vi "ResMgr-BackgroundThread.vi"(7 "Name (Unnamed)":string) -> ()   [LabVIEW 2017, in "Communicable State Machine.lvlib"]
uses:
  Communicable State Machine.lvlib
  Typedef/_CSM_GlobalLog_MSG.ctl
  Typedef/_CSM_Response Source Message.ctl
  Typedef/_CSM_GlobalLog_MSG_TYPE.ctl
  CSMQ/_CSMObj-ModeData.ctl
  CSMQ/_CSMObj-Data.ctl
  Typedef/_CSM_MSG_TYPE.ctl
  Priority Queue/Priority Queue.ctl
  Typedef/_Cross CSM State Data.ctl
  Typedef/_Cross CSM State Response.ctl
  Priority Queue/def-Data(LowPRI-Q).ctl
  Typedef/_CSM Status Change Event Data.ctl
panel:
  out "Array":string[](array[string])
  out "size(s)":i32
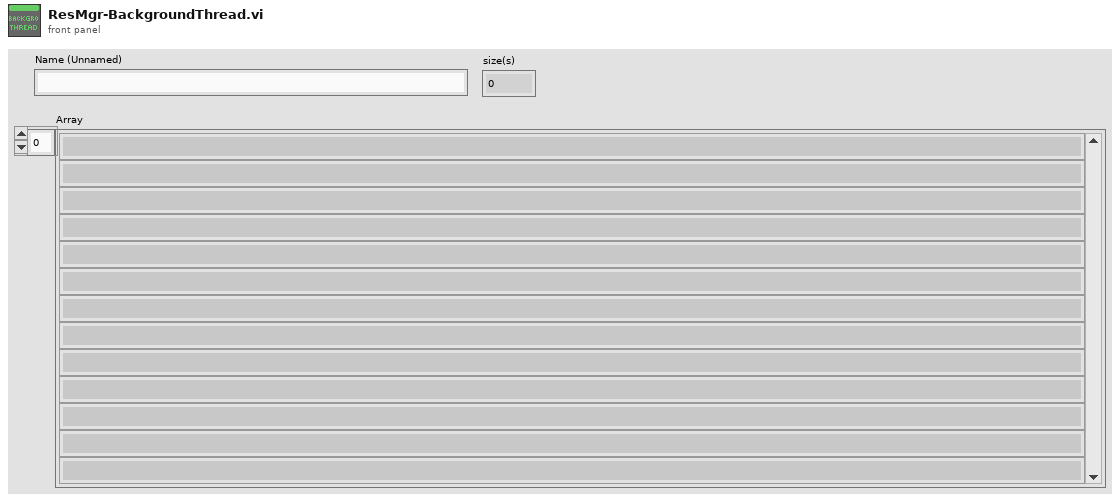
[diagram p1: front panel]
types:
  T1 = typedef "Communicable State Machine.lvlib/_CSM_GlobalLog_MSG.ctl" = cluster{"Name (\"\" to Use UUID)":string, "Current State":string, "Arguments":string, "Source Message":T2, "Source Module":string, "Complete(T)/Start(F)":bool, "LogType":T3, "Time Stamp":timestamp}
  T2 = typedef "Communicable State Machine.lvlib/_CSM_Response Source Message.ctl" = cluster{"‘State":string, "’Arguments":string, "’Error":errorcluster}
  T3 = typedef "Communicable State Machine.lvlib/_CSM_GlobalLog_MSG_TYPE.ctl" = enum16{"User Log", "State Change", "Status", "Interrupt", "Register", "Unregister", "Error Log", "Module Created", "Module Destroyed", "Async Message", "No-Rep Async Message", "Sync Message"}
  T4 = typedef "Communicable State Machine.lvlib/_CSMObj-ModeData.ctl" = cluster{"CSMDataDVR":refnum<data-value>[], "PriorityQueues":T5[], "Messages of Chain Nodes":cluster{"Module Name":string, "Allowed Messages":string[]}[], "Chain Message Mapping Map":variant, "SharedRegistryRules":string[]}
  T5 = typedef "Communicable State Machine.lvlib/Priority Queue.ctl" = cluster{"HPriorityQ":refnum<queue>, "LowPriorityQ":refnum<queue>}
  T6 = typedef "Communicable State Machine.lvlib/_CSM Status Change Event Data.ctl" = cluster{"ModuleName":string, "Status":string, "Arguments":string}
  T7 = cluster{"ResType":string, "RespQ":refnum<queue>, "Parameter":string, "WatchDogQ":refnum<queue>}
  T8 = cluster{"Major":u16, "Minor":u16, "Fix":u16, "Build":u16}
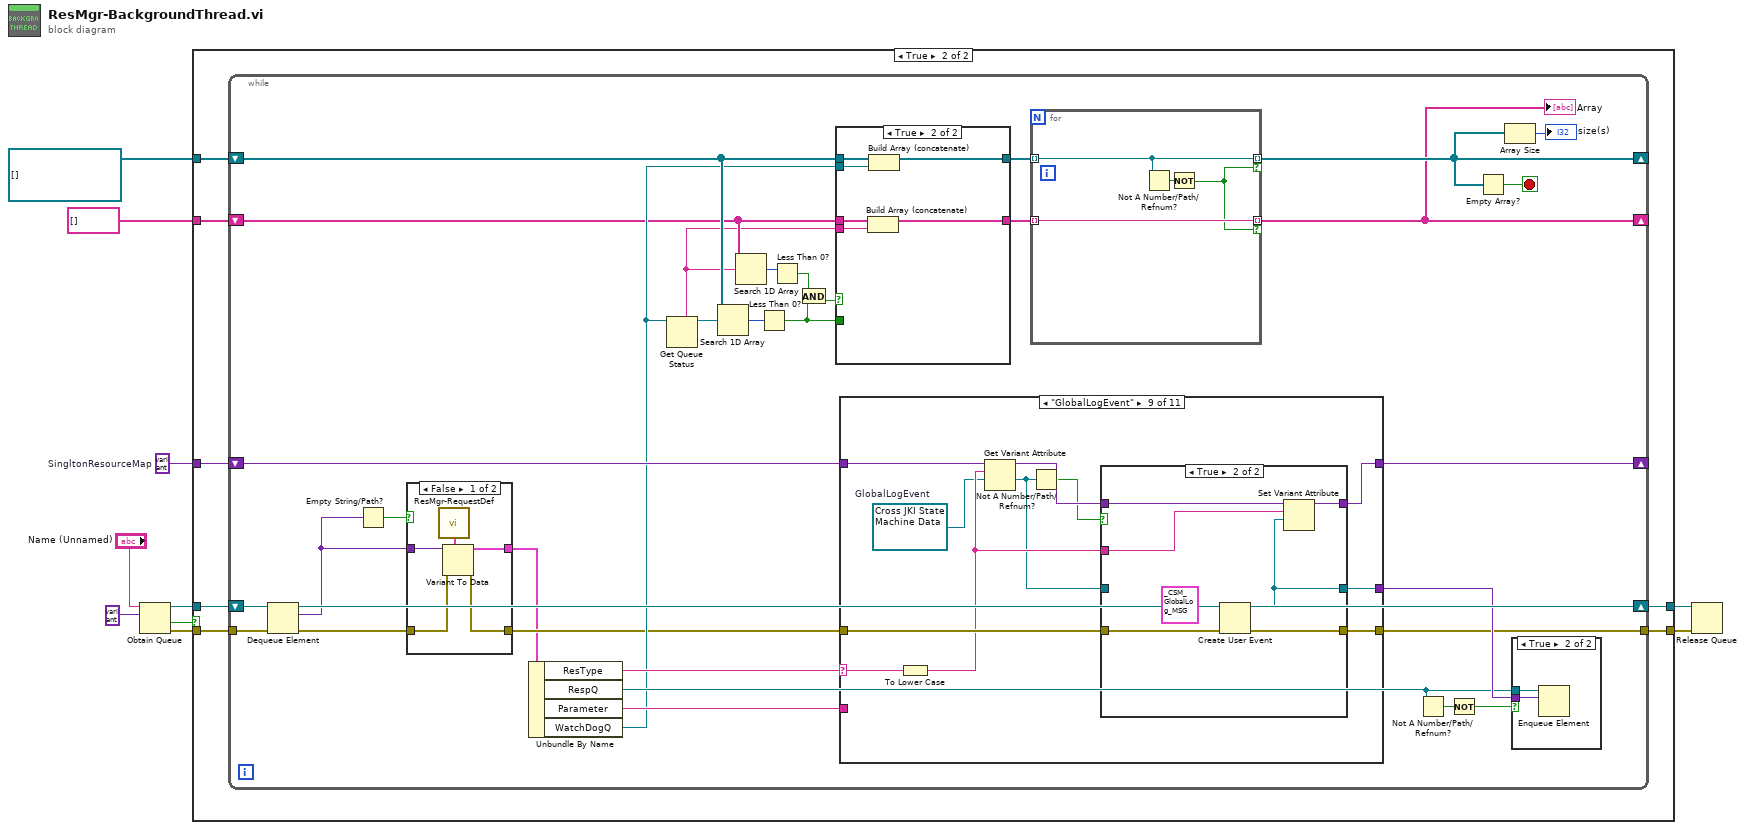
[diagram p0: block diagram]
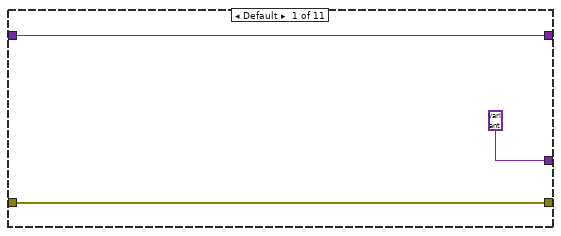
[diagram p6: hidden frame]
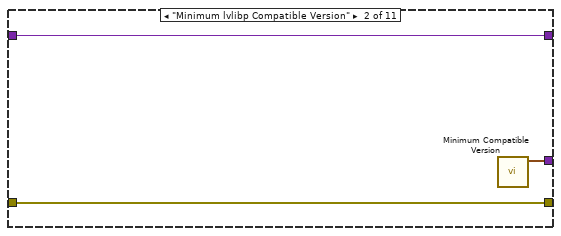
[diagram p7: hidden frame]
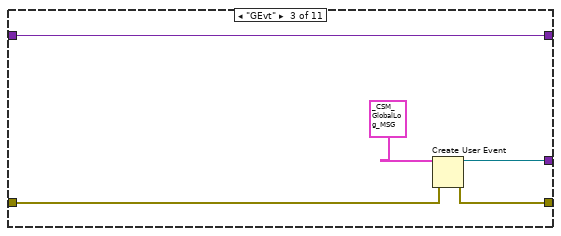
[diagram p8: hidden frame]
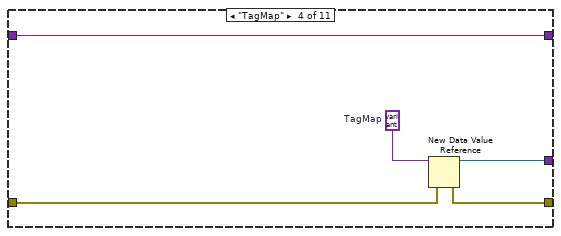
[diagram p9: hidden frame]
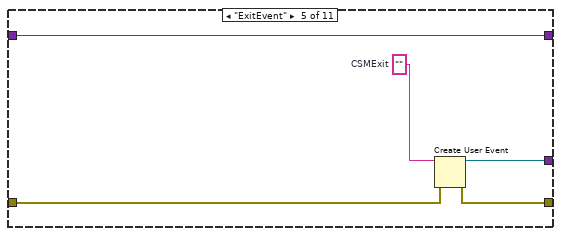
[diagram p10: hidden frame]
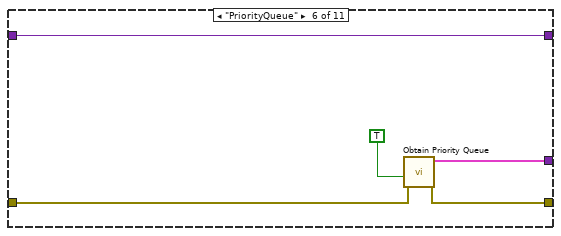
[diagram p11: hidden frame]
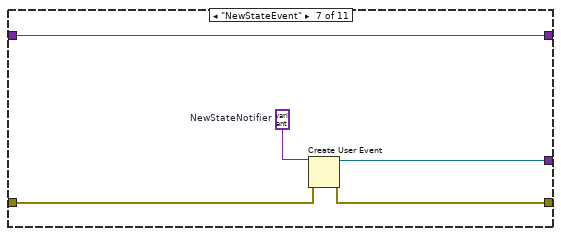
[diagram p12: hidden frame]
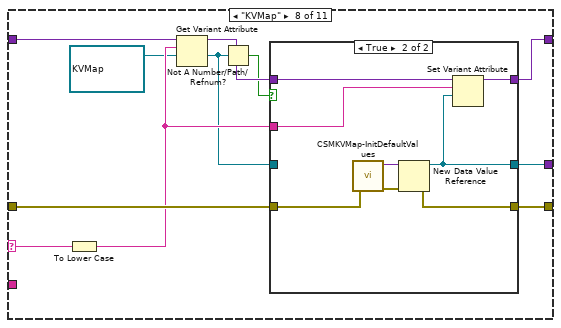
[diagram p13: hidden frame]
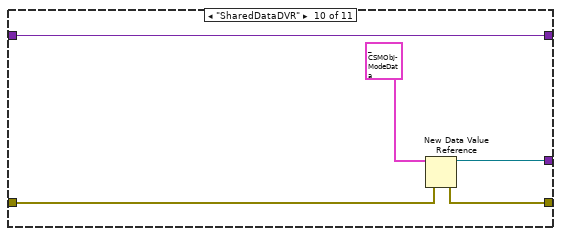
[diagram p16: hidden frame]
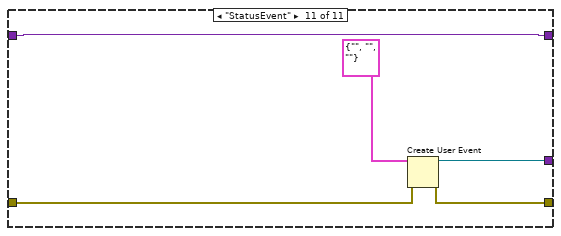
[diagram p17: hidden frame]
diagram:
  w4 = variant  # SingltonResourceMap
  n1 = Obtain Queue(name (unnamed)="Name (Unnamed)", element data type=variant) -> (queue out=w10:refnum<queue>, created new?=w3:bool, error out=w9:errorcluster)  [unwired: 3 in]
  n2 = case shown="True" w3 {
    tunnel: w10 -> [w12 w19]
    tunnel: w9 -> [w11 w18]
    tunnel: [w12 w17] -> w8
    tunnel: [w11 w16] -> w7
    tunnel: refnum<queue>[] [] ("WatchDogQ") -> [_ w15]
    tunnel: w4 -> [_ w14]
    tunnel: string[] [] ("WatchDogQ") -> [_ w13]
    frame False {
    }
    frame True {
      n3 = while {
        tunnel: w18 -> [w51]
        shift-right: [w49] -> w17
        shift-left: w19 -> [w52]
        tunnel: [w46] -> w16
        shift-right: [w34] -> _
        shift-left: w15 -> [w39]
        shift-right: [w36] -> _
        shift-left: w14 -> [w35]
        shift-right: [w30] -> _
        shift-left: w13 -> [w29]
        stop <- w43 stop-if-true
        n4 = Dequeue Element(queue=w52, error in (no error)=w51) -> (queue out=w49:refnum<queue>, element=w21:variant, error out=w48:errorcluster)  [unwired: 1 in, 1 out]
        n5 = Empty String/Path?(string/path=w21) -> (empty?=w20:bool)
        n6 = case shown="False" w20 {
          tunnel: w48 -> [w57 w58]
          tunnel: [w56 w58] -> w23
          tunnel: [w54 _] -> w22
          tunnel: w21 -> [w53 _]
          frame False {
            n7 = call "ResMgr-RequestDef.vi"() -> ("ResMgr-RequestDef.ctl"=w55:T7)  [unwired: 2 in]
            n8 = Variant To Data(error in=w57, type=w55, Variant=w53) -> (data=w54:T7, error out=w56:errorcluster)
          }
          frame True {
          }
        }
        n9 = Unbundle By Name(w22) -> ("ResType"=w50:string, "RespQ"=w41:refnum<queue>, "Parameter"=w45:string, "WatchDogQ"=w33:refnum<queue>)
        n10 = Get Queue Status(queue=w33) -> (queue out=w32:refnum<queue>, queue name=w28:string)  [unwired: 2 in, 6 out]
        n11 = Search 1D Array(1D array=w39, element=w32) -> (index of element=w38:i32)  [unwired: 1 in]
        n12 = Search 1D Array(1D array=w29, element=w28) -> (index of element=w27:i32)  [unwired: 1 in]
        n13 = Less Than 0?(x=w38) -> (x < 0?=w24:bool)
        n14 = Less Than 0?(x=w27) -> (x < 0?=w25:bool)
        n15 = And(x=w25, y=w24) -> (x .and. y?=w26:bool)
        n16 = case shown="True" w26 {
          tunnel: [w60 w64] -> w44
          tunnel: w39 -> [w60 w66]
          tunnel: w33 -> [_ w65]
          tunnel: w29 -> [w59 w63]
          tunnel: w28 -> [_ w62]
          tunnel: [w59 w61] -> w31
          tunnel: w24 -> [_ _]
          frame False {
          }
          frame True {
            n17 = Build Array (concatenate)(w63, w62) -> (w61:string[])
            n18 = Build Array (concatenate)(w66, w65) -> (w64:refnum<queue>[])
          }
        }
        n19 = case shown="\"GlobalLogEvent\"" w50 {
          selector: w50 -> [_ _ _ _ _ _ _ w110 w132 _ _]
          tunnel: [variant w76 w82 w86 w90 w97 w102 w107 w129 w148 w155] -> w47
          tunnel: w23 -> [w75 w78 w80 w85 w92 w95 w100 w113 w135 w149 w153]
          tunnel: [w75 w78 w81 w87 w91 w96 w101 w114 w136 w150 w154] -> w46
          tunnel: w45 -> [_ _ _ _ _ _ _ _ _ _ _]
          tunnel: [w73 w77 w79 w84 w89 w94 w99 w109 w131 w147 w152] -> w36
          tunnel: w35 -> [w73 w77 w79 w84 w89 w94 w99 w112 w134 w147 w152]
          frame Default {
          }
          frame "Minimum lvlibp Compatible Version" {
            n20 = call "Minimum Compatible Version.vi"() -> ("Min-Compatible Version"=w76:T8)  [unwired: 10 in, 1 out]
          }
          frame "GEvt" {
            n21 = Create User Event(user event datatype=T1 {"Name (\"\" to Use UUID)"="", "Current State"="", "Arguments"="", "Source Message"={"‘State"="", "’Arguments"="", "’Error"={"status"=FALSE, "code"=0, "source"=""}}, "Source Module"="", "Complete(T)/Start(F)"=FALSE, "LogType"=enum."State Change", "Time Stamp"=timestamp(0 s since 1904-01-01)} ("Cross JKI State Machine Data"), error in=w80) -> (user event=w82:refnum<user-event>, error out=w81:errorcluster)
          }
          frame "TagMap" {
            w88 = variant  # TagMap
            n22 = New Data Value Reference(data value=w88, error in=w85) -> (data value reference=w86:refnum<data-value>, error out=w87:errorcluster)
          }
          frame "ExitEvent" {
            w93 = ""  # CSMExit
            n23 = Create User Event(user event datatype=w93, error in=w92) -> (user event=w90:refnum<user-event>, error out=w91:errorcluster)
          }
          frame "PriorityQueue" {
            n24 = call "Obtain Priority Queue.vi"("error in (no error)"=w95, "Create If Not Found? (T)"=TRUE ("create if not found? (T)")) -> ("error out"=w96:errorcluster, "Priority Queue"=w97:T5)  [unwired: 7 in, 1 out]
          }
          frame "NewStateEvent" {
            w103 = variant  # NewStateNotifier
            n25 = Create User Event(user event datatype=w103, error in=w100) -> (user event=w102:refnum<user-event>, error out=w101:errorcluster)
          }
          frame "KVMap" {
            n26 = To Lower Case(string=w110) -> (all lower case string=w108:string)
            n27 = Get Variant Attribute(Variant=w112, name=w108, default value (empty Variant)=refnum<data-value> refnum ("data value reference")) -> (duplicate Variant=w111:variant, value=w104:refnum<data-value>)  [unwired: 1 in, 2 out]
            n28 = Not A Number/Path/Refnum?(number/path/refnum=w104) -> (NaN/Path/Refnum?=w105:bool)
            n29 = case shown="True" w105 {
              tunnel: [w116 w125] -> w114
              tunnel: w113 -> [w116 w118]
              tunnel: w111 -> [w115 w124]
              tunnel: [w115 w123] -> w109
              tunnel: w108 -> [_ w122]
              tunnel: [w117 w121] -> w107
              tunnel: w104 -> [w117 _]
              frame False {
              }
              frame True {
                n30 = call "CSMKVMap-InitDefaultValues.vi"("error in"=w118) -> ("error out"=w119:errorcluster, "KVMap"=w120:variant)  [unwired: 9 in]
                n31 = New Data Value Reference(data value=w120, error in=w119) -> (data value reference=w121:refnum<data-value>, error out=w125:errorcluster)
                n32 = Set Variant Attribute(Variant=w124, name=w122, value=w121) -> (Variant out=w123:variant)  [unwired: 1 in, 2 out]
              }
            }
          }
          frame "GlobalLogEvent" {
            w126 = refnum<user-event> refnum  # GlobalLogEvent
            n33 = To Lower Case(string=w132) -> (all lower case string=w130:string)
            n34 = Get Variant Attribute(Variant=w134, name=w130, default value (empty Variant)=w126) -> (duplicate Variant=w133:variant, value=w127:refnum<user-event>)  [unwired: 1 in, 2 out]
            n35 = Not A Number/Path/Refnum?(number/path/refnum=w127) -> (NaN/Path/Refnum?=w128:bool)
            n36 = case shown="True" w128 {
              tunnel: [w138 w141] -> w136
              tunnel: w135 -> [w138 w142]
              tunnel: w133 -> [w137 w146]
              tunnel: [w137 w145] -> w131
              tunnel: w130 -> [_ w144]
              tunnel: [w139 w140] -> w129
              tunnel: w127 -> [w139 _]
              frame False {
              }
              frame True {
                n37 = Create User Event(user event datatype=T1 {"Name (\"\" to Use UUID)"="", "Current State"="", "Arguments"="", "Source Message"={"‘State"="", "’Arguments"="", "’Error"={"status"=FALSE, "code"=0, "source"=""}}, "Source Module"="", "Complete(T)/Start(F)"=FALSE, "LogType"=enum."State Change", "Time Stamp"=timestamp(0 s since 1904-01-01)} ("Cross JKI State Machine Data"), error in=w142) -> (user event=w140:refnum<user-event>, error out=w141:errorcluster)
                n38 = Set Variant Attribute(Variant=w146, name=w144, value=w140) -> (Variant out=w145:variant)  [unwired: 1 in, 2 out]
              }
            }
          }
          frame "SharedDataDVR" {
            n39 = New Data Value Reference(data value=T4 {"CSMDataDVR"=[], "PriorityQueues"=[], "Messages of Chain Nodes"=[], "Chain Message Mapping Map"=variant, "SharedRegistryRules"=[]} ("CSMObj-Data"), error in=w149) -> (data value reference=w148:refnum<data-value>, error out=w150:errorcluster)
          }
          frame "StatusEvent" {
            n40 = Create User Event(user event datatype=T6 {"ModuleName"="", "Status"="", "Arguments"=""} ("Status Message"), error in=w153) -> (user event=w155:refnum<user-event>, error out=w154:errorcluster)
          }
        }
        n41 = for {
          tunnel: w44 -> [w70] mode=indexing
          tunnel: [w70] -> w34 mode=indexing if=w67
          tunnel: [w68] -> w30 mode=indexing if=w67
          tunnel: w31 -> [w68] mode=indexing
          n42 = Not A Number/Path/Refnum?(number/path/refnum=w70) -> (NaN/Path/Refnum?=w69:bool)
          n43 = Not(x=w69) -> (.not. x?=w67:bool)
        }
        "Array" <- w30
        n44 = Not A Number/Path/Refnum?(number/path/refnum=w41) -> (NaN/Path/Refnum?=w42:bool)
        n45 = Not(x=w42) -> (.not. x?=w40:bool)
        n46 = Empty Array?(array=w34) -> (empty?=w43:bool)
        n47 = Array Size(array=w34) -> (size(s)=→"size(s)":i32)
        n48 = case shown="True" w40 {
          tunnel: w47 -> [_ w72]
          tunnel: w41 -> [_ w71]
          frame False {
          }
          frame True {
            n49 = Enqueue Element(queue=w71, element=w72) -> ()  [unwired: 2 in, 3 out]
          }
        }
      }
    }
  }
  n50 = Release Queue(queue=w8, error in (no error)=w7) -> ()  [unwired: 1 in, 3 out]
